vi "PH_SRDG645.PC Set Output.vi"(0 "i ref in":refnum<vi>, 1 "Output to set":T1 items=["T0", "AB", "CD", "EF", "GH"], 2 "Output Settings":T2={"Level Offset [V]"=0.0, "Amplitue [V]"=1000.0, "Polarity"=0} {"Polarity" items=["negative", "positive"]}, 5 "error IO":errorcluster) -> (14 "i ref out":refnum<vi>, 17 "Something changed?":bool, 19 "error out":errorcluster)   [LabVIEW 2014, in "PH_SRDG645.lvlib"]
doc: "This VI communicates with the hardware to set the output settings."
uses:
  PH_SRDG645.lvlib
  instr.lib/Stanford Research DG645/Driver/Output BNC.ctl
  instr.lib/Stanford Research DG645/Stanford Research DG645 - Driver.lvlib
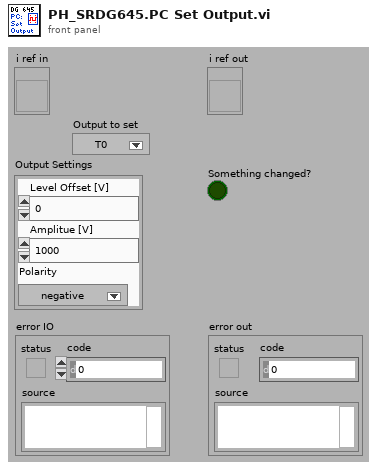
[diagram p1: front panel]
types:
  T1 = typedef "Stanford Research DG645 - Driver.lvlib/Output BNC.ctl" = i32
  T2 = cluster{"Level Offset [V]":dbl, "Amplitue [V]":dbl, "Polarity":i32}
  T3 = typedef "PH_SRDG645.lvlib/PH_SRDG645.i attribute.ctl" = cluster{"GUI Refs":cluster{"Delete":refnum<vi>, "Device Errors":refnum<vi>, "Trigger":refnum<vi>, "Default Name":refnum<vi>, "Firmware Revision":refnum<vi>, "Serial Number":refnum<vi>, "Model":refnum<vi>, "Visa resource name":refnum<vi>}, "Service ID Rate":i32, "Service IDs Channelinfo":i32[], "VISA resource name":refnum<visa-resource-name>, "Device Errors":cluster{"code":i32, "Text":string}[], "Trigger":T4, "Channels":cluster{"T1":T5, "A":T5, "B":T5, "C":T5, "D":T5, "E":T5, "F":T5, "G":T5, "H":T5}, "GUI Refs Channels":refnum<vi>[], "Outputs":cluster{"AB":cluster{"Level Offset [V]":dbl, "Amplitue [V]":dbl, "Polarity":i32}, "CD":cluster{"Level Offset [V]":dbl, "Amplitue [V]":dbl, "Polarity":i32}, "EF":cluster{"Level Offset [V]":dbl, "Amplitue [V]":dbl, "Polarity":i32}, "GH":cluster{"Level Offset [V]":dbl, "Amplitue [V]":dbl, "Polarity":i32}, "T0":cluster{"Level Offset [V]":dbl, "Amplitue [V]":dbl, "Polarity":i32}}, "GUI Refs Outputs":refnum<vi>[], "Serial Number":string, "Firmweare Revision":string, "Model":string}
  T4 = typedef "PH_SRDG645.lvlib/PH_SRDG645.Trigger.ctl" = cluster{"Source":i32, "Rate [Hz]":dbl, "Level [V]":dbl}
  T5 = typedef "PH_SRDG645.lvlib/PH_SRDG645.Channel Settings.ctl" = cluster{"Delay [s]":dbl, "relative to":i32}
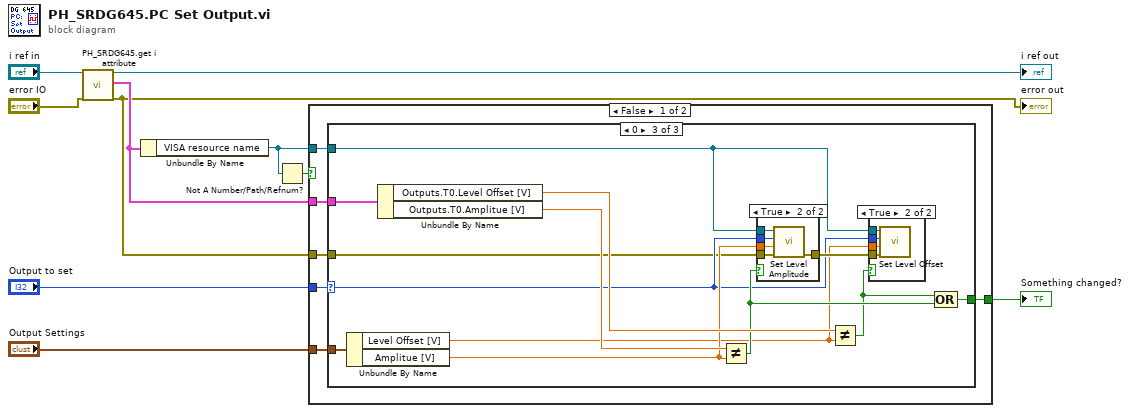
[diagram p0: block diagram]
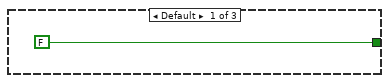
[diagram p2: hidden frame]
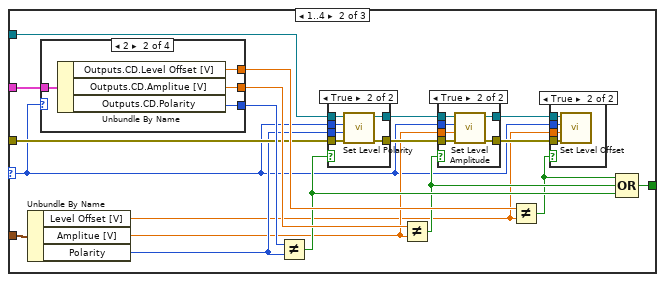
[diagram p3: hidden frame]
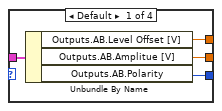
[diagram p4: hidden frame]
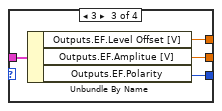
[diagram p5: hidden frame]
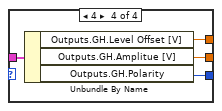
[diagram p6: hidden frame]
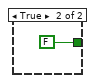
[diagram p12: hidden frame]
diagram:
  n1 = call "PH_SRDG645.get i attribute.vi"("i ref in"="i ref in", "error in (no error)"="error IO") -> ("i ref out"=→"i ref out":refnum<vi>, "i attribute"=w4:T3, "error out"=w1:errorcluster)  [unwired: 15 in]
  "error out" <- w1
  n2 = Unbundle By Name(w4) -> ("VISA resource name"=w2:refnum<visa-resource-name>)
  n3 = Not A Number/Path/Refnum?(number/path/refnum=w2) -> (NaN/Path/Refnum?=w3:bool)
  n4 = case shown="False" w3 {
    tunnel: "Output Settings" -> [w16 _]
    tunnel: w1 -> [w15 _]
    tunnel: [w14 FALSE] -> w6
    tunnel: "Output to set" -> [w13 _]
    tunnel: w4 -> [w12 _]
    tunnel: w2 -> [w11 _]
    frame False {
      n5 = case shown="0" w13 {
        selector: w13 -> [_ w21 w75]
        tunnel: w12 -> [_ w36 w85]
        tunnel: w16 -> [_ w35 w84]
        tunnel: w15 -> [_ w30 w74]
        tunnel: [FALSE w32 w81] -> w14
        tunnel: w11 -> [_ w18 w73]
        frame Default {
        }
        frame 1..4 {
          n6 = Unbundle By Name(w35) -> ("Level Offset [V]"=w23:dbl, "Amplitue [V]"=w25:dbl, "Polarity"=w28:i32)
          n7 = case shown="2" w21 {
            tunnel: w36 -> [w40 w44 w48 w52]
            tunnel: [w39 w43 w47 w51] -> w34
            tunnel: [w38 w42 w46 w50] -> w33
            tunnel: [w37 w41 w45 w49] -> w31
            frame Default {
              n8 = Unbundle By Name(w40) -> ("Outputs.AB.Level Offset [V]"=w38:dbl, "Outputs.AB.Amplitue [V]"=w39:dbl, "Outputs.AB.Polarity"=w37:i32)
            }
            frame 2 {
              n9 = Unbundle By Name(w44) -> ("Outputs.CD.Level Offset [V]"=w42:dbl, "Outputs.CD.Amplitue [V]"=w43:dbl, "Outputs.CD.Polarity"=w41:i32)
            }
            frame 3 {
              n10 = Unbundle By Name(w48) -> ("Outputs.EF.Level Offset [V]"=w46:dbl, "Outputs.EF.Amplitue [V]"=w47:dbl, "Outputs.EF.Polarity"=w45:i32)
            }
            frame 4 {
              n11 = Unbundle By Name(w52) -> ("Outputs.GH.Level Offset [V]"=w50:dbl, "Outputs.GH.Amplitue [V]"=w51:dbl, "Outputs.GH.Polarity"=w49:i32)
            }
          }
          n12 = Not Equal?(x=w31, y=w28) -> (x != y?=w29:bool)
          n13 = case shown="True" w29 {
            tunnel: w30 -> [w66 w72]
            tunnel: [w66 w71] -> w27
            tunnel: w21 -> [_ w70]
            tunnel: w28 -> [_ w69]
            tunnel: w18 -> [w65 w68]
            tunnel: [w65 w67] -> w20
            frame False {
            }
            frame True {
              n14 = call "Set Level Polarity.vi"("error in (no error)"=w72, "Polarity (positive)"=w69, "Output BNC (AB)"=w70, "VISA resource name"=w68) -> ("error out"=w71:errorcluster, "VISA resource name out"=w67:refnum<visa-resource-name>)  [unwired: 5 in, 1 out]
            }
          }
          n15 = Not Equal?(x=w34, y=w25) -> (x != y?=w26:bool)
          n16 = case shown="True" w26 {
            tunnel: w27 -> [w58 w64]
            tunnel: [w58 w63] -> w24
            tunnel: w20 -> [w57 w62]
            tunnel: w25 -> [_ w61]
            tunnel: w21 -> [_ w60]
            tunnel: [w57 w59] -> w19
            frame False {
            }
            frame True {
              n17 = call "Set Level Amplitude.vi"("error in (no error)"=w64, "Level Amplitude (0) [V]"=w61, "Output BNC (T0)"=w60, "VISA resource name"=w62) -> ("error out"=w63:errorcluster, "VISA resource name out"=w59:refnum<visa-resource-name>)  [unwired: 5 in, 1 out]
            }
          }
          n18 = Not Equal?(x=w33, y=w23) -> (x != y?=w22:bool)
          n19 = case shown="True" w22 {
            tunnel: w24 -> [_ w56]
            tunnel: w19 -> [_ w55]
            tunnel: w23 -> [_ w54]
            tunnel: w21 -> [_ w53]
            frame False {
            }
            frame True {
              n20 = call "Set Level Offset.vi"("error in (no error)"=w56, "Level Offset (0) [V]"=w54, "Output BNC (T0)"=w53, "VISA resource name"=w55) -> ()  [unwired: 5 in, 3 out]
            }
          }
          n21 = Compound Arithmetic op=OR(w22, w26, w29) -> (w32:bool)
        }
        frame 0 {
          n22 = Unbundle By Name(w84) -> ("Level Offset [V]"=w77:dbl, "Amplitue [V]"=w79:dbl)
          n23 = Unbundle By Name(w85) -> ("Outputs.T0.Level Offset [V]"=w82:dbl, "Outputs.T0.Amplitue [V]"=w83:dbl)
          n24 = Not Equal?(x=w83, y=w79) -> (x != y?=w80:bool)
          n25 = case shown="True" w80 {
            tunnel: w74 -> [w90 w95]
            tunnel: [w90 w94] -> w78
            tunnel: w73 -> [_ w93]
            tunnel: w79 -> [_ w92]
            tunnel: w75 -> [_ w91]
            frame False {
            }
            frame True {
              n26 = call "Set Level Amplitude.vi"("error in (no error)"=w95, "Level Amplitude (0) [V]"=w92, "Output BNC (T0)"=w91, "VISA resource name"=w93) -> ("error out"=w94:errorcluster)  [unwired: 5 in, 2 out]
            }
          }
          n27 = Not Equal?(x=w82, y=w77) -> (x != y?=w76:bool)
          n28 = case shown="True" w76 {
            tunnel: w78 -> [_ w89]
            tunnel: w73 -> [_ w88]
            tunnel: w77 -> [_ w87]
            tunnel: w75 -> [_ w86]
            frame False {
            }
            frame True {
              n29 = call "Set Level Offset.vi"("error in (no error)"=w89, "Level Offset (0) [V]"=w87, "Output BNC (T0)"=w86, "VISA resource name"=w88) -> ()  [unwired: 5 in, 3 out]
            }
          }
          n30 = Compound Arithmetic op=OR(w76, w80) -> (w81:bool)
        }
      }
    }
    frame True {
    }
  }
  "Something changed?" <- w6
